vi "LoadConnectionID.vi"(8 "ArrayIN":T1(array[cluster])=[{"IPaddress"="127.0.0.1", "Port"=63400, "connection ID"=refnum, "TCP error"={"status"=TRUE, "code"=1, "source"="TCP Write in TCPwrite8bytesMC.vi->PicoCmdClientMOVE-ForMasterControl_3.vi->Manual command_11.vi"}}], 10 "Port":i32, 11 "IPaddress":string) -> (0 "ArrayOUT":T1(array[cluster])=[{"IPaddress"="127.0.0.1", "Port"=63400, "connection ID"=refnum, "TCP error"={"status"=TRUE, "code"=1, "source"="TCP Write in TCPwrite8bytesMC.vi->PicoCmdClientMOVE-ForMasterControl_3.vi->Manual command_11.vi"}}], 1 "index":i32, 2 "ConnectError":errorcluster, 3 "connection ID":refnum<k5>)   [LabVIEW 2013]
panel:
  out "Status":bool=TRUE
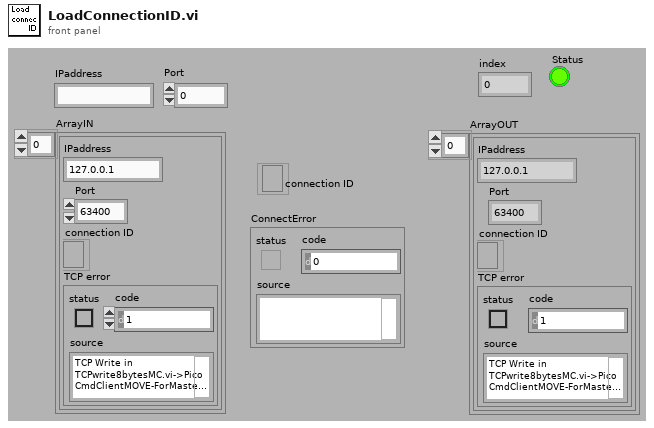
[diagram p1: front panel]
types:
  T1 = cluster{"IPaddress":string, "Port":i32, "connection ID":refnum<k5>, "TCP error":errorcluster}[]
  T2 = cluster{"IPaddress":string, "Port":i32, "connection ID":refnum<k5>, "ConnectError":errorcluster}
  T3 = cluster{"IPaddress":string, "Port":i32, "connection ID":refnum<k5>, "ConnectError":errorcluster}[]
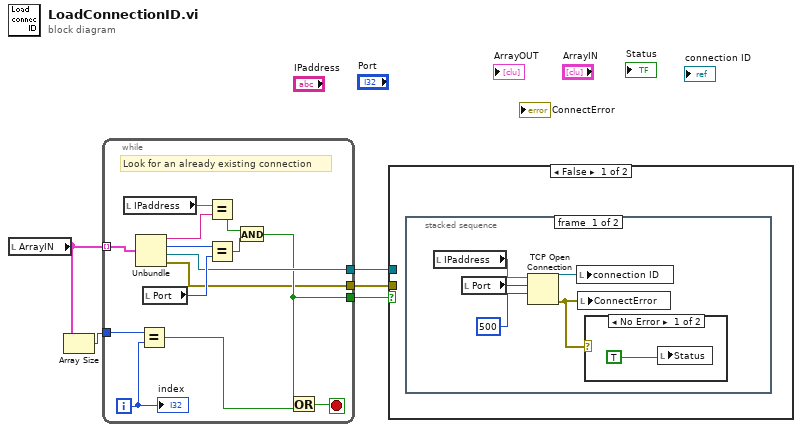
[diagram p0: block diagram]
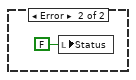
[diagram p2: hidden frame]
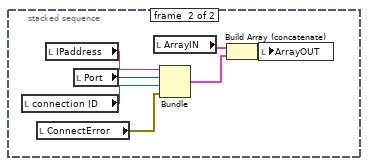
[diagram p3: hidden frame]
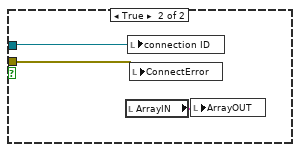
[diagram p4: hidden frame]
diagram:
  n1 = local read "ArrayIN"() -> (w5:T1)
  n2 = Array Size(array=w5) -> (size(s)=w4:i32)
  n3 = while {
    tunnel: w5 -> [w19] mode=indexing
    tunnel: w4 -> [w17]
    tunnel: [w8] -> w3
    tunnel: [w7] -> w2
    tunnel: [w6] -> w1
    i -> [w18]
    stop <- w16 stop-if-true
    # "Look for an already existing connection"
    n4 = local read "IPaddress"() -> (w13:string)
    n5 = Unbundle(w19) -> ("IPaddress"=w14:string, "Port"=w12:i32, "connection ID"=w8:refnum<k5>, "TCP error"=w6:errorcluster)
    n6 = Equal?(x=w17, y=w18) -> (x = y?=w15:bool)
    n7 = local read "Port"() -> (w11:i32)
    n8 = Equal?(x=w13, y=w14) -> (x = y?=w10:bool)
    n9 = Equal?(x=w12, y=w11) -> (x = y?=w9:bool)
    n10 = And(x=w10, y=w9) -> (x .and. y?=w7:bool)
    n11 = Or(x=w7, y=w15) -> (x .or. y?=w16:bool)
    "index" <- w18
  }
  n12 = case shown="False" w2 {
    tunnel: w3 -> [_ w36]
    tunnel: w1 -> [_ w34]
    frame False {
      n13 = stacked-sequence {
        frame #0 {
          n14 = local read "IPaddress"() -> (w24:string)
          n15 = local read "Port"() -> (w23:i32)
          n16 = TCP Open Connection(address=w24, remote port or service name=w23, timeout ms (60000)=500) -> (connection ID=w21:refnum<k5>, error out=w20:errorcluster)  [unwired: 1 in, 1 out]
          n17 = local write "connection ID"(w21) -> ()
          n18 = local write "ConnectError"(w20) -> ()
          n19 = case shown="No Error" w20 {
            frame No Error {
              n20 = local write "Status"(TRUE) -> ()
            }
            frame Error {
              n21 = local write "Status"(FALSE ("Error")) -> ()
            }
          }
        }
        frame #1 {
          n22 = local read "connection ID"() -> (w31:refnum<k5>)
          n23 = local read "ConnectError"() -> (w27:errorcluster)
          n24 = local read "IPaddress"() -> (w33:string)
          n25 = local read "Port"() -> (w32:i32)
          n26 = local read "ArrayIN"() -> (w30:T1)
          n27 = Bundle("IPaddress"=w33, "Port"=w32, "connection ID"=w31, "ConnectError"=w27) -> (w28:T2)  [unwired: 1 out]
          n28 = Build Array (concatenate)(w30, w28) -> (w29:T3)
          n29 = local write "ArrayOUT"(w29) -> ()
        }
      }
    }
    frame True {
      n30 = local read "ArrayIN"() -> (w35:T1)
      n31 = local write "connection ID"(w36) -> ()
      n32 = local write "ConnectError"(w34) -> ()
      n33 = local write "ArrayOUT"(w35) -> ()
    }
  }
